vi "hw3.1.vi"() -> (3 "Array 3":dbl[](array[numeric]))   [LabVIEW 2014]
panel:
  out "Waveform Graph":dbl[](graph)
  out "subarray":dbl[](array[numeric])
  out "Array":dbl[](array[numeric])
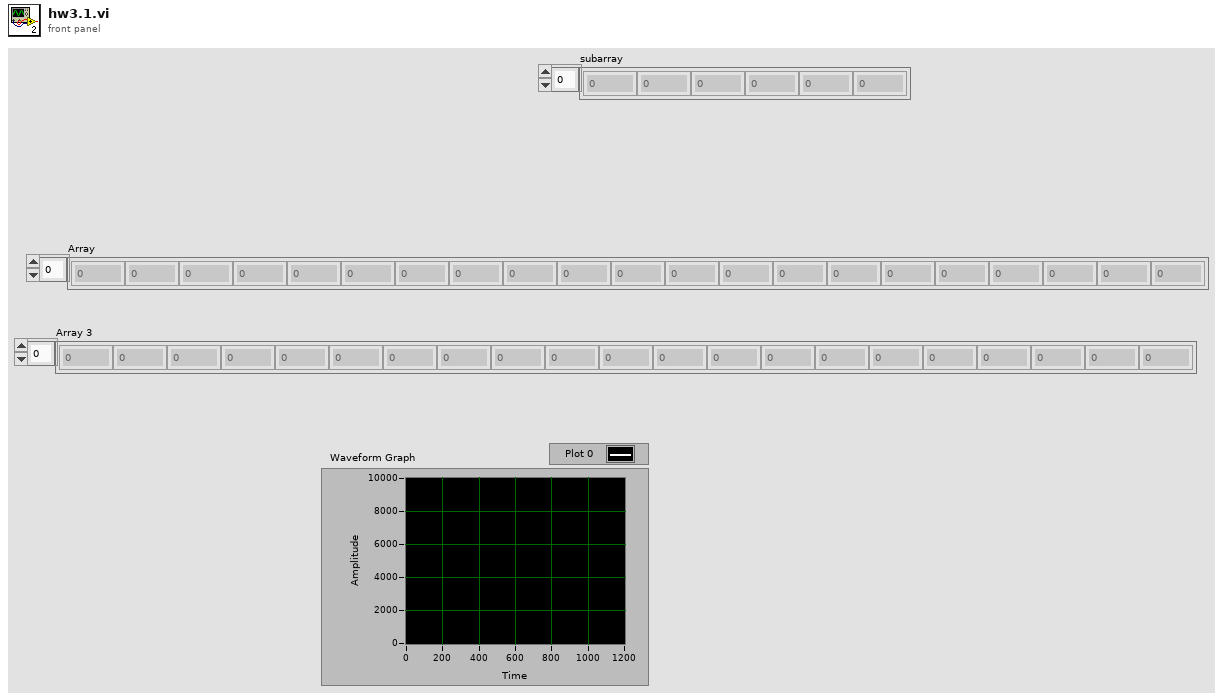
[diagram p1: front panel]
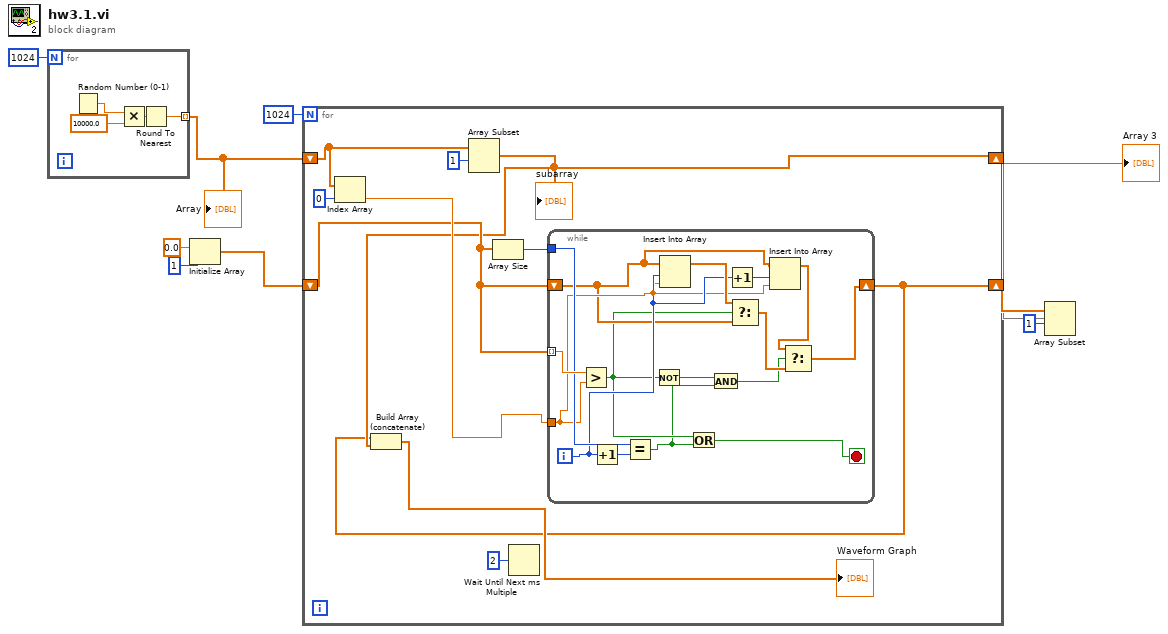
[diagram p0: block diagram]
diagram:
  n1 = for {
    N: 1024 -> [_]
    tunnel: [w10] -> w3 mode=indexing
    n2 = Random Number (0-1)() -> (number: 0 to 1=w13:dbl)
    n3 = Multiply(x=w13, y=10000.0) -> (x*y=w11:dbl)
    n4 = Round To Nearest(number=w11) -> (nearest integer value=w10:dbl)
  }
  "Array" <- w3
  n5 = Initialize Array(0.0 ("element"), 1 ("dimension size")) -> (w6:dbl[])
  n6 = for {
    N: 1024 -> [_]
    shift-right: [w14] -> w9
    shift-left: w6 -> [w18]
    shift-right: [w15] -> _
    shift-left: w3 -> [w17]
    n7 = Index Array(array=w17, index=0) -> (element=w22:dbl)
    n8 = Array Subset(array=w17, index=1) -> (w15:dbl[])  [unwired: 1 in]
    "subarray" <- w15
    n9 = Array Size(array=w18) -> (size(s)=w23:i32)
    n10 = Wait Until Next ms Multiple(millisecond multiple=u32 2) -> ()  [unwired: 1 out]
    n11 = while {
      tunnel: w18 -> [w39] mode=indexing
      tunnel: w23 -> [w38]
      shift-right: [w28] -> w14
      shift-left: w18 -> [w30]
      tunnel: w22 -> [w32]
      i -> [w34]
      stop <- w36 stop-if-true
      n12 = Greater?(x=w39, y=w32) -> (0:w27:bool)
      n13 = Increment(x=w34) -> (x+1=w37:i32)
      n14 = Equal?(x=w38, y=w37) -> (x = y?=w26:bool)
      n15 = Not(x=w27) -> (.not. x?=w25:bool)
      n16 = Insert Into Array(array=w30, index=w34, new element=w32) -> (w35:dbl[])
      n17 = Or(x=w27, y=w26) -> (x .or. y?=w36:bool)
      n18 = And(x=w25, y=w26) -> (x .and. y?=w24:bool)
      n19 = Increment(x=w34) -> (x+1=w33:i32)
      n20 = Select(t=w35, s=w27, f=w30) -> (s? t:f=w29:dbl[])
      n21 = Insert Into Array(array=w30, index=w33, new element=w32) -> (w31:dbl[])
      n22 = Select(t=w31, s=w24, f=w29) -> (s? t:f=w28:dbl[])
    }
    n23 = Build Array (concatenate)(w14, w15) -> (→"Waveform Graph":dbl[])
  }
  n24 = Array Subset(array=w9, index=1) -> (→"Array 3":dbl[])  [unwired: 1 in]
